vi "rqcAlice ServiceNET Check Connection.vi"(8 "error in":errorcluster, 11 "rqcAlice ServiceNET in":T1) -> (0 "error out":errorcluster, 3 "rqcAlice ServiceNET out":T1)   [LabVIEW 2019]
uses:
  Custom Controls/rqcAlice ServiceNET control.ctl
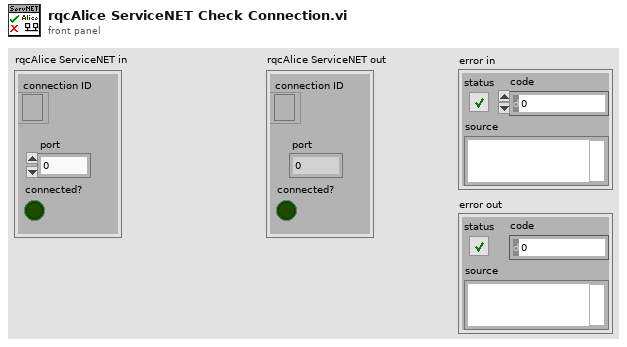
[diagram p1: front panel]
types:
  T1 = typedef "rqcAlice ServiceNET control.ctl" = cluster{"connection ID":refnum<k5>, "port":u16, "connected?":bool}
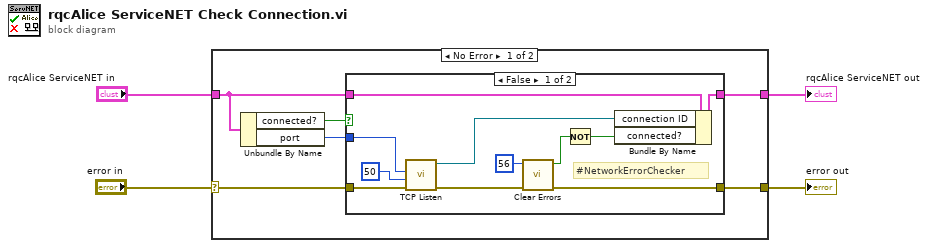
[diagram p0: block diagram]
diagram:
  n1 = case shown="No Error" "error in" {
    selector: "error in" -> [w6 w25]
    tunnel: [w5 w25] -> w3
    tunnel: "rqcAlice ServiceNET in" -> [w9 w24]
    tunnel: [w8 w24] -> w1
    frame No Error {
      n2 = Unbundle By Name(w9) -> ("connected?"=w10:bool, "port"=w7:u16)
      n3 = case shown="False" w10 {
        tunnel: [w20 w23] -> w8
        tunnel: w9 -> [w21 w23]
        tunnel: w7 -> [w19 _]
        tunnel: w6 -> [w18 w22]
        tunnel: [w14 w22] -> w5
        frame False {
          # "#NetworkErrorChecker"
          n4 = call <vilib>:"TCP Listen.vi"("error in (no error)"=w18, "timeout ms (wait forever: -1)"=50, "port"=w19) -> ("error out"=w15:errorcluster, "connection ID"=w17:refnum<k5>)  [unwired: 4 in, 3 out]
          n5 = call <vilib>:"Clear Errors.vi"("error in (no error)"=w15, "specific error code to clear (0: all)"=56) -> ("error out"=w14:errorcluster, "specific error cleared?"=w12:bool)  [unwired: 4 in]
          n6 = Not(x=w12) -> (.not. x?=w13:bool)
          n7 = Bundle By Name(cluster=w21, "connection ID"=w17, "connected?"=w13) -> (w20:T1)
        }
        frame True {
        }
      }
    }
    frame Error {
    }
  }
  "rqcAlice ServiceNET out" <- w1
  "error out" <- w3
